vi "Handle MissionOp Deploy AIP.vi"(8 "error in (no error)":errorcluster, 11 "RDS Mission Controller Actor in":refnum<class "RDS Mission Controller Actor.lvclass">) -> (0 "error out":errorcluster, 3 "RDS Mission Controller Actor out":refnum<class "RDS Mission Controller Actor.lvclass">)   [LabVIEW 2015, in "RDS Mission Controller Actor.lvlib" / "RDS Mission Controller Actor.lvclass"]
uses:
  RDS Mission Controller Actor.lvclass
  Libraries/RDS Framework/RDS Message Class/AIP Command Control.ctl
  AIP Instrument/AIP Instrument.lvlib
  Libraries/RDS Child Messages/RDS Child Messages.lvlib
  Actors/RDS Parent Actor/RDS Parent Actor/RDS Parent Actor.lvclass
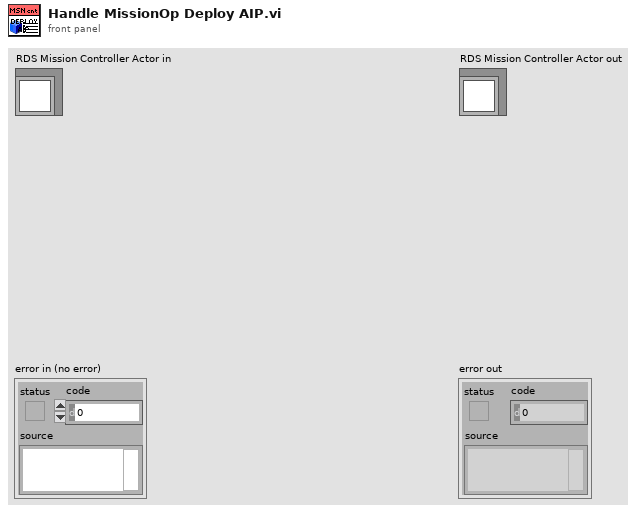
[diagram p1: front panel]
types:
  T1 = typedef "RDS Child Messages.lvlib/AIP Command Control.ctl" = enum16{"Stow", "Deploy", "Stop", "Validate Sensors", "Jog Deploy FP", "Jog Stow FP", "Jog Deploy FS", "Jog Stow FS", "Jog Deploy AP", "Jog Stow AP", "Jog Deploy AS", "Jog Stow AS", "Deploy FP", "Deploy FS", "Deploy AP", "Deploy AS", "Stow FP", "Stow FS", "Stow AP", "Stow AS"}
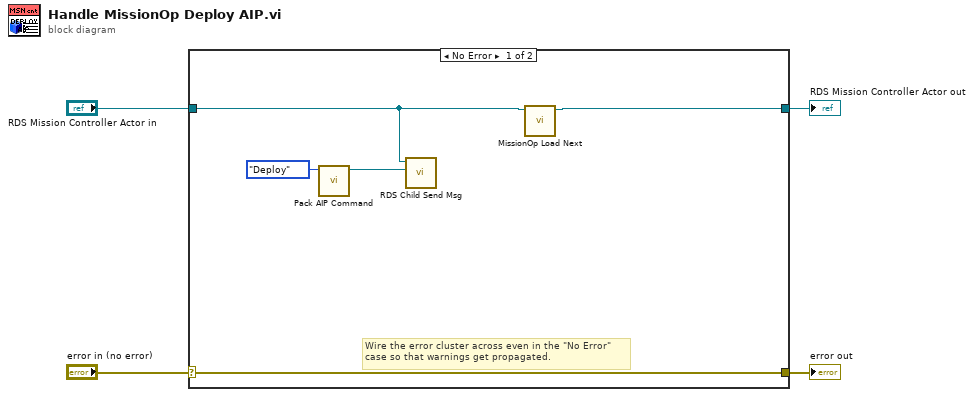
[diagram p0: block diagram]
diagram:
  n1 = case shown="No Error" "error in (no error)" {
    selector: "error in (no error)" -> [w9 w11]
    tunnel: [w9 w11] -> w3
    tunnel: [w5 w10] -> w1
    tunnel: "RDS Mission Controller Actor in" -> [w6 w10]
    frame No Error {
      # "Wire the error cluster across even in the \"No Error\"\ncase so that warnings get propagated."
      n2 = call "Pack AIP Command.vi"("AIP Command"=AIP_Command_Control."Deploy") -> ("AIP Deploy Command out"=w7:refnum<class "AIP Command.lvclass">)  [unwired: 10 in]
      n3 = call "RDS Child Send Msg.vi"("RDS Message"=w7, "RDS Parent Actor in"=w6) -> ()  [unwired: 8 in, 2 out]
      n4 = call "MissionOp Load Next.vi"("RDS Mission Controller Actor in"=w6) -> ("RDS Mission Controller Actor out"=w5:refnum<class "RDS Mission Controller Actor.lvclass">)  [unwired: 9 in, 1 out]
    }
    frame Error {
    }
  }
  "error out" <- w3
  "RDS Mission Controller Actor out" <- w1
